vi "DisplayDataChartDialog.vi"(8 "Error In":errorcluster) -> (0 "Error Out":errorcluster)   [LabVIEW 2012]
uses:
  DisplayDataChartAction.ctl
  <vilib>/Platform/TimedLoop/XDataNode/timing_clust.ctl
  <vilib>/Platform/TimedLoop/XDataNode/nitl_modes.ctl
  <vilib>/Platform/TimedLoop/XDataNode/wakeup.ctl
  DisplayDataGlobalAction.ctl
  <vilib>/platform/TimedLoop/XDataNode/XDataNode.xnode
  <vilib>/Platform/TimedLoop/XDataNode/XDNodeRunTimeDep.lvlib
panel:
  in  "RESET":bool
  in  "Live DUT":u32=1 min=1 step=1
  in  "Live SMU":enum16{"A", "B"}(ring)
  in  "Live Measure Value":enum16{"Voltage", "Current", "Resistance"}(ring)
  out "Live SMU Value":dbl format="%_4p"
  out "Live SMU Units":enum16{"V", "A", "Ohm"}(ring)
  out "Live SMU Chart":dbl(graph)
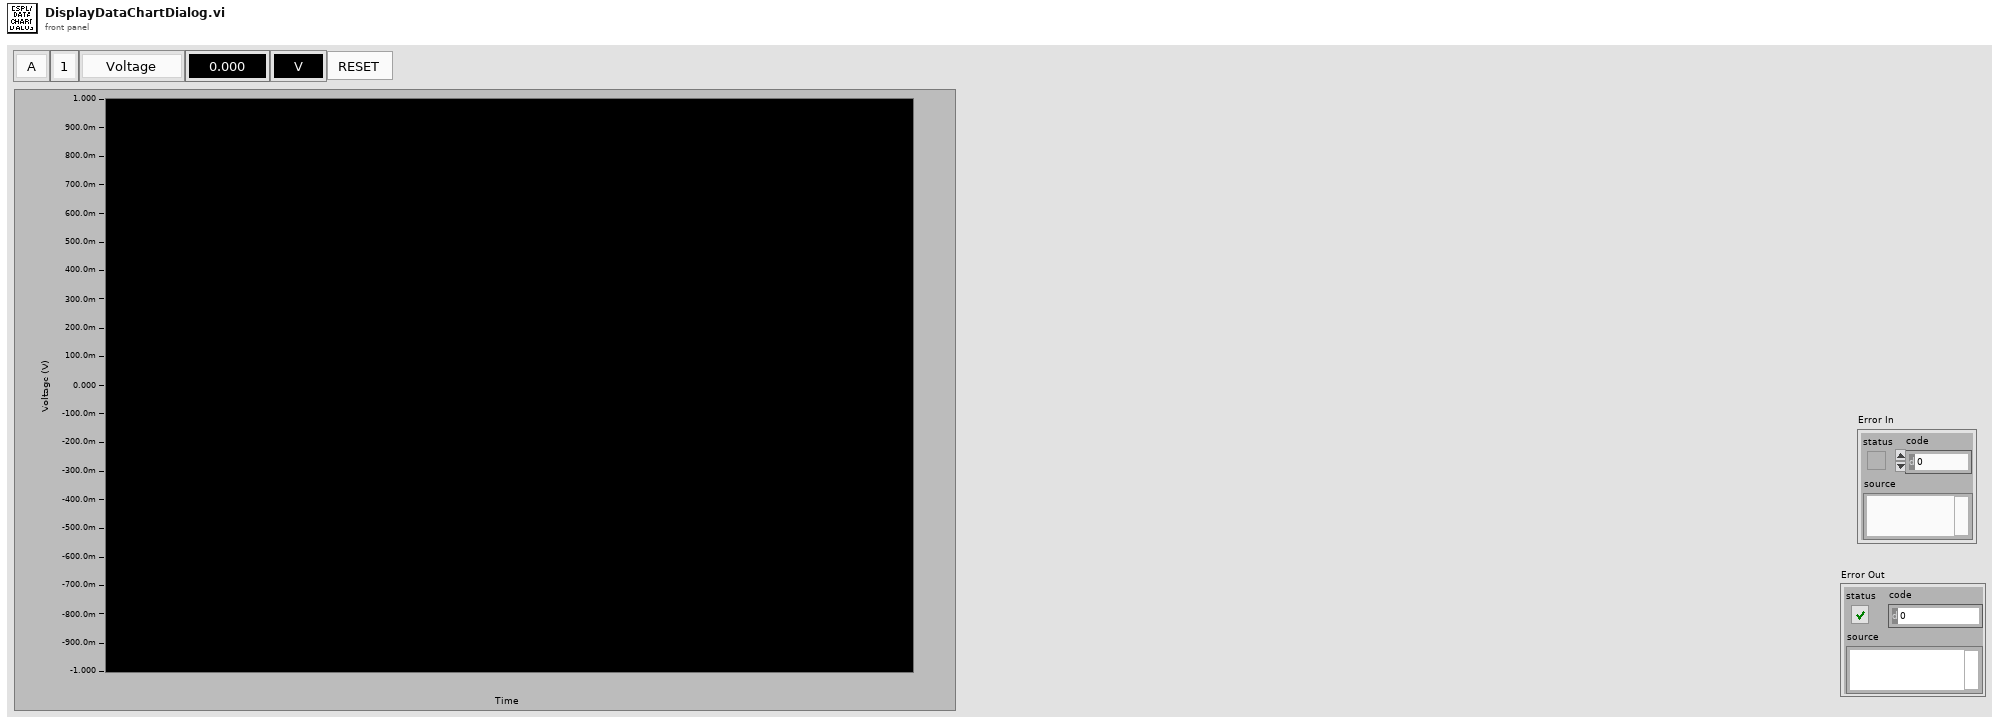
[diagram p1: front panel]
types:
  T1 = typedef "DisplayDataGlobalAction.ctl" = enum16{"Get", "Set"}
  T2 = typedef "XDNodeRunTimeDep.lvlib/timing_clust.ctl" = cluster{"Expected End [f-1]":u64, "Actual End [f-1]":u64, "Finished Late? [f-1]":bool, "Expected End [i-1]":u64, "Actual End [i-1]":u64, "Finished Late? [i-1]":bool, "Expected Start [i]":u64, "Actual Start [i]":u64, "Expected Start [f]":u64, "Actual Start [f]":u64, "Source Name":string, "Structure Name":string, "Period":i64, "Deadline":i64, "Offset":i64, "Start":i64, "Priority":i32, "Timeout":i32, "Mode":T3, "Wakeup Reason":T4, "Error":errorcluster, "Source Type":string, "Secondary Source Type":string, "Global End Time":u64, "Global Start Time":u64, "Frame Duration":u64, "Iteration Duration":u64, "Assigned CPU":i32, "I/O Scan Engine Mode":u32}
  T3 = typedef "XDNodeRunTimeDep.lvlib/nitl_modes.ctl" = enum32{"No Change", "Process missed periods, maintain original phase", "Discard missed periods, maintain original phase", "Process missed periods, ignore original phase", "Discard missed periods, ignore original phase"}
  T4 = typedef "XDNodeRunTimeDep.lvlib/wakeup.ctl" = enum32{"Normal", "Aborted", "Asynchronous wakeup", "Timing source error", "Timed loop error", "Timeout"}
  T5 = typedef "DisplayDataChartAction.ctl" = enum16{"Initialize", "Shutdown", "Update", "Reset"}
  T6 = cluster{"Live SMU":enum16{"A", "B"}, "Live DUT":u32, "Live Measure Value":enum16{"Voltage", "Current", "Resistance"}}
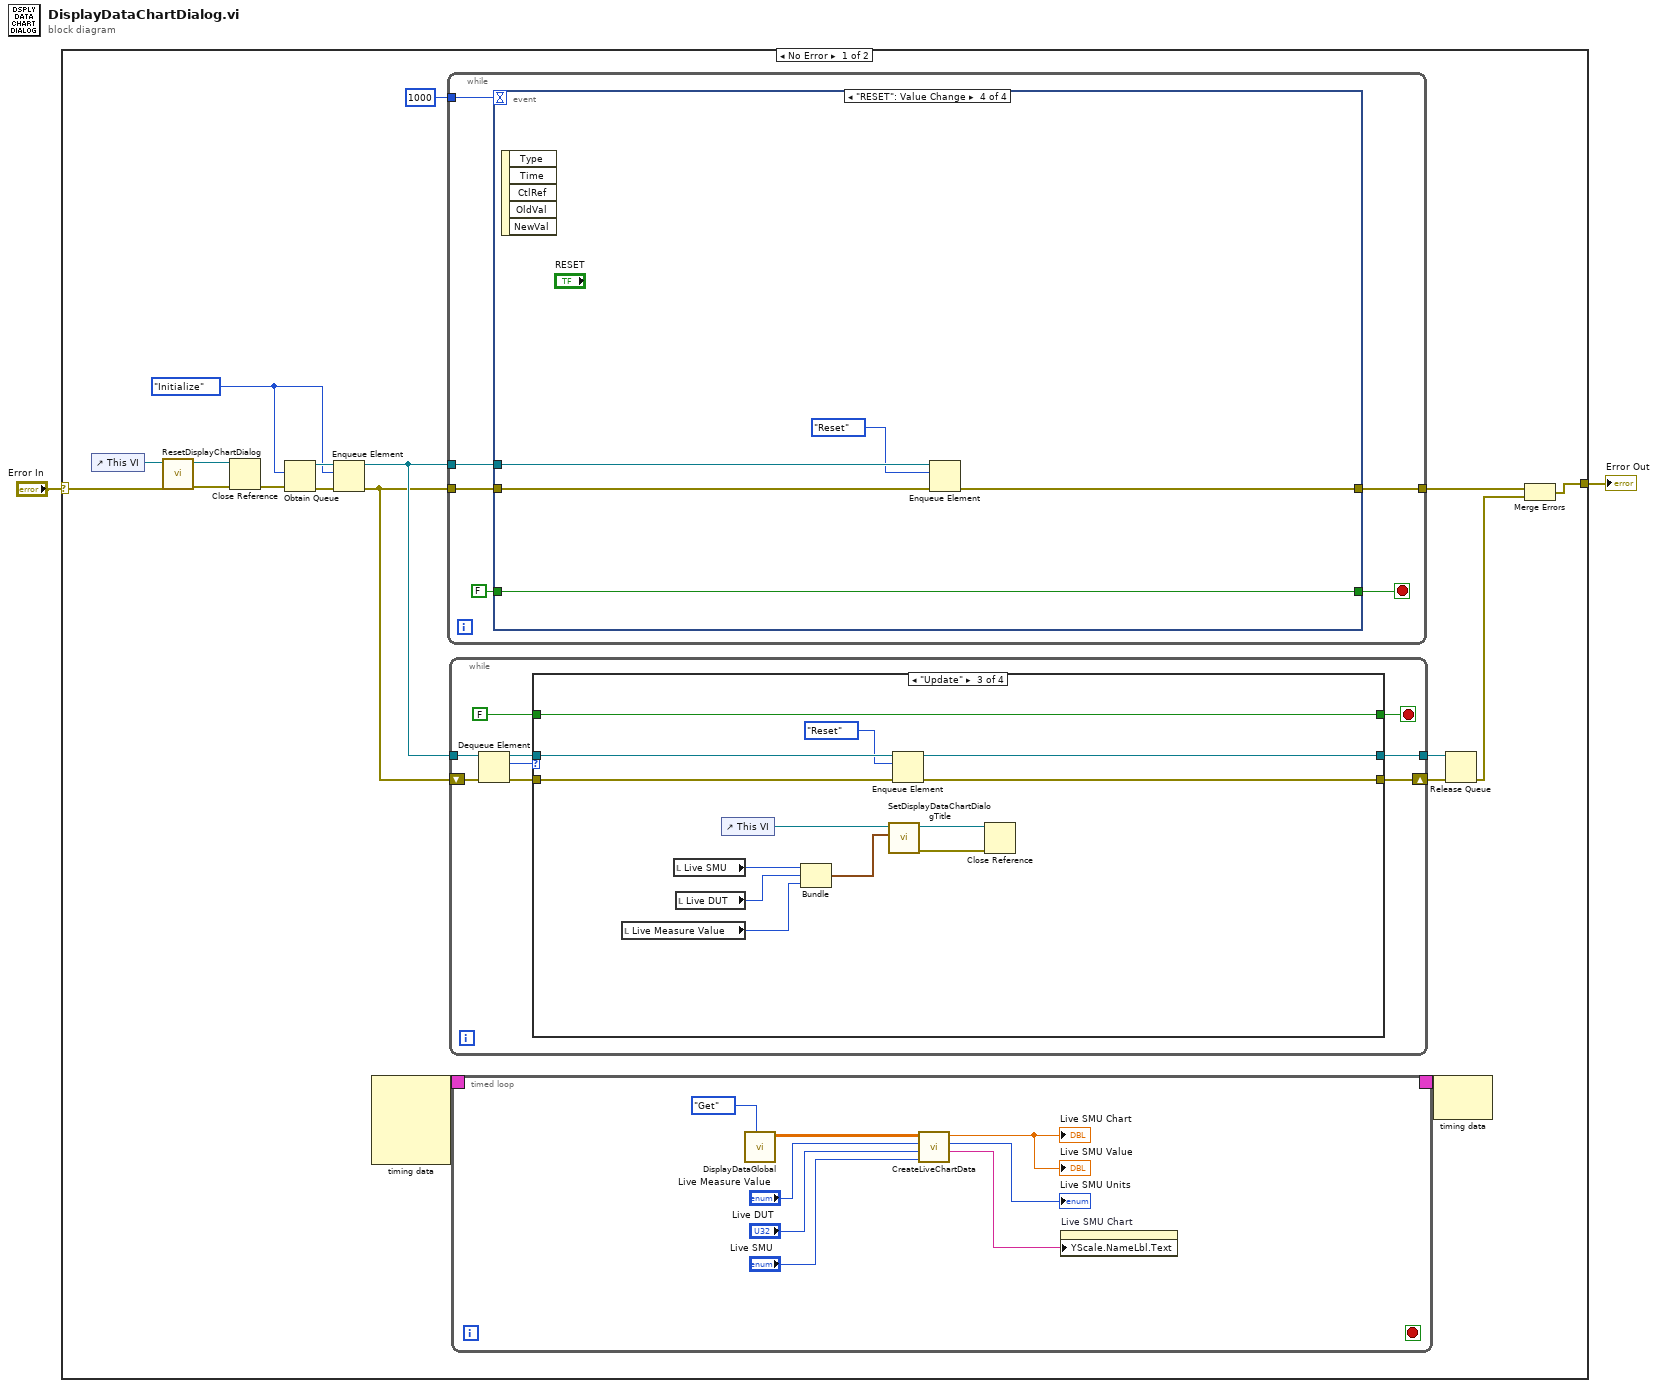
[diagram p0: block diagram]
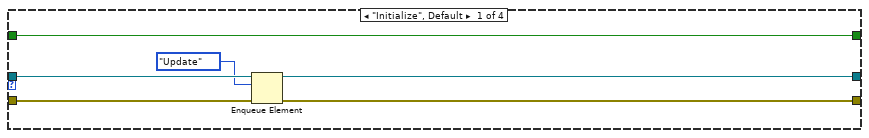
[diagram p2: hidden frame]
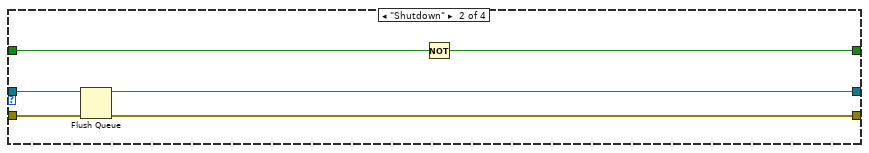
[diagram p3: hidden frame]
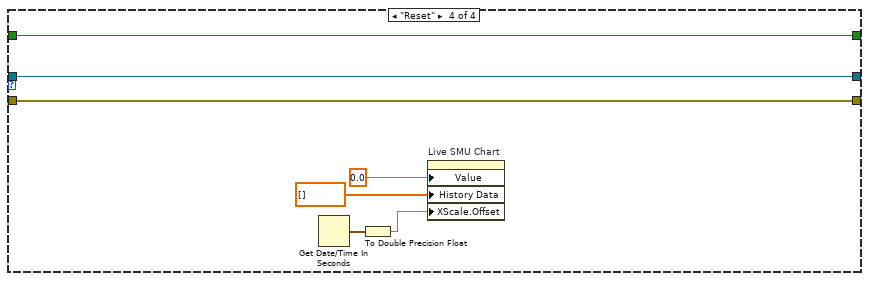
[diagram p4: hidden frame]
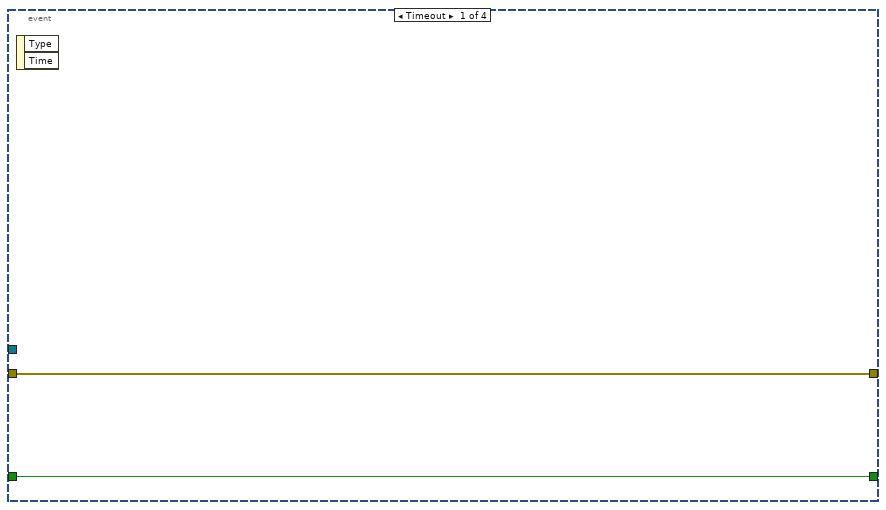
[diagram p5: hidden frame]
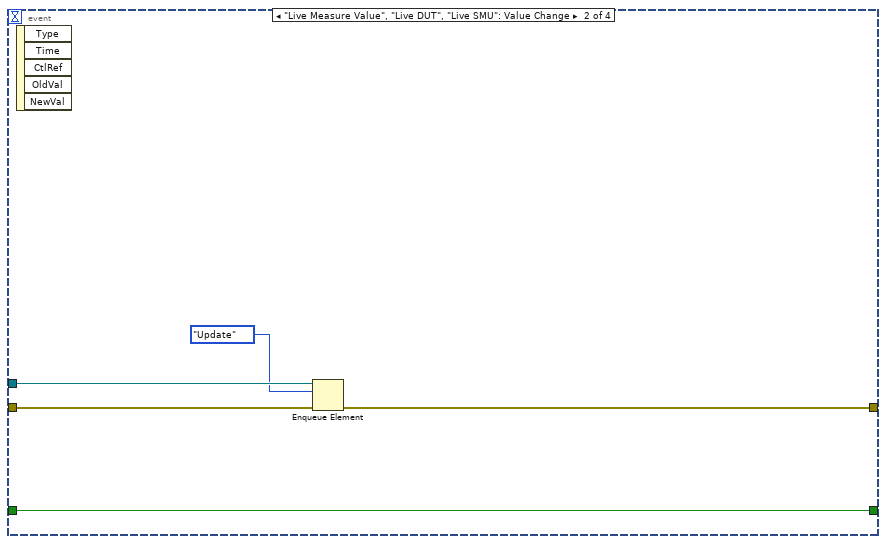
[diagram p6: hidden frame]
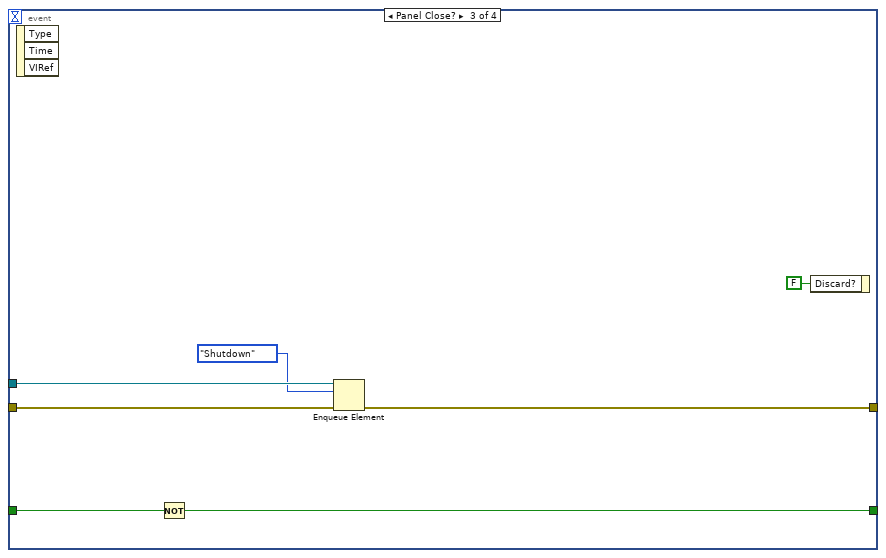
[diagram p7: hidden frame]
diagram:
  n1 = case shown="No Error" "Error In" {
    selector: "Error In" -> [w3 w99]
    tunnel: [w11 w99] -> w1
    frame No Error {
      w15 = DisplayDataChartAction."Initialize" ("Action")
      n2 = control-ref of="This VI"() -> (w4:refnum<vi>)
      n3 = call "ResetDisplayChartDialog.vi"("Error In"=w3, "VI Ref In"=w4) -> ("Error Out"=w6:errorcluster, "VI Ref Out"=w7:refnum<vi>)  [unwired: 8 in]
      n4 = Close Reference(reference=w7, error in (no error)=w6) -> (error out=w5:errorcluster)
      n5 = Obtain Queue(element data type=w15, error in (no error)=w5) -> (queue out=w17:refnum<queue>, error out=w16:errorcluster)  [unwired: 3 in, 1 out]
      n6 = Enqueue Element(queue=w17, element=w15, error in (no error)=w16) -> (queue out=w14:refnum<queue>, error out=w13:errorcluster)  [unwired: 1 in, 1 out]
      n7 = node-c288() -> (w19:T2)  [unwired: 4 in]
      n8 = while {
        tunnel: 1000 -> [w77]
        tunnel: w14 -> [w76]
        tunnel: w13 -> [w75]
        tunnel: [w74] -> w12
        stop <- w78 stop-if-true
        n9 = event shown="[3] \"RESET\": Value Change" {
          selector: _ -> [_ _ _ _]
          dyn-events: _ -> [_ _ _ _]
          timeout: w77 -> [_ _ _ _]
          tunnel: FALSE -> [w81 w86 w90 w98]
          tunnel: [w81 w86 w89 w98] -> w78
          tunnel: w76 -> [_ w84 w92 w95]
          tunnel: w75 -> [w80 w85 w91 w97]
          tunnel: [w80 w82 w88 w96] -> w74
          event Timeout {
            n10 = event-data() -> ()  [unwired: 1 in, 2 out]
          }
          event "Live Measure Value", "Live DUT", "Live SMU": Value Change {
            n11 = event-data() -> ()  [unwired: 1 in, 5 out]
            n12 = Enqueue Element(queue=w84, element=DisplayDataChartAction."Update", error in (no error)=w85) -> (error out=w82:errorcluster)  [unwired: 1 in, 2 out]
          }
          event Panel Close? {
            n13 = event-data() -> ()  [unwired: 1 in, 3 out]
            n14 = Not(x=w90) -> (.not. x?=w89:bool)
            n15 = Enqueue Element(queue=w92, element=DisplayDataChartAction."Shutdown", error in (no error)=w91) -> (error out=w88:errorcluster)  [unwired: 1 in, 2 out]
            n16 = event-data("Discard?"=FALSE) -> ()  [unwired: 1 in, 1 out]
          }
          event "RESET": Value Change {
            n17 = event-data() -> ()  [unwired: 1 in, 5 out]
            n18 = Enqueue Element(queue=w95, element=DisplayDataChartAction."Reset", error in (no error)=w97) -> (error out=w96:errorcluster)  [unwired: 1 in, 2 out]
          }
        }
      }
      n19 = while {
        tunnel: w14 -> [w39]
        shift-right: [w34] -> w9
        shift-left: w13 -> [w38]
        tunnel: [w33] -> w10
        stop <- w40 stop-if-true
        n20 = Dequeue Element(queue=w39, error in (no error)=w38) -> (queue out=w36:refnum<queue>, element=w37:T5, error out=w35:errorcluster)  [unwired: 1 in, 1 out]
        n21 = case shown="\"Update\"" w37 {
          tunnel: FALSE -> [w47 w53 w66 w68]
          tunnel: [w47 w52 w66 w68] -> w40
          tunnel: w36 -> [w46 w51 w65 w67]
          tunnel: w35 -> [w45 w50 w64 w69]
          tunnel: [w44 w49 w63 w69] -> w34
          tunnel: [w42 w48 w61 w67] -> w33
          frame "Initialize", Default {
            n22 = Enqueue Element(queue=w46, element=DisplayDataChartAction."Update", error in (no error)=w45) -> (queue out=w42:refnum<queue>, error out=w44:errorcluster)  [unwired: 1 in, 1 out]
          }
          frame "Shutdown" {
            n23 = Flush Queue(queue=w51, error in (no error)=w50) -> (queue out=w48:refnum<queue>, error out=w49:errorcluster)  [unwired: 1 out]
            n24 = Not(x=w53) -> (.not. x?=w52:bool)
          }
          frame "Update" {
            n25 = local read "Live Measure Value"() -> (w55:enum16{"Voltage", "Current", "Resistance"})
            n26 = local read "Live SMU"() -> (w57:enum16{"A", "B"})
            n27 = local read "Live DUT"() -> (w56:u32)
            n28 = control-ref of="This VI"() -> (w60:refnum<vi>)
            n29 = Bundle("Live SMU"=w57, "Live DUT"=w56, "Live Measure Value"=w55) -> (w54:T6)  [unwired: 1 in]
            n30 = call "SetDisplayDataChartDialogTitle.vi"("Chart Settings"=w54, "VI Ref In"=w60) -> ("Error Out"=w58:errorcluster, "VI Ref Out"=w59:refnum<vi>)  [unwired: 8 in]
            n31 = Enqueue Element(queue=w65, element=DisplayDataChartAction."Reset", error in (no error)=w64) -> (queue out=w61:refnum<queue>, error out=w63:errorcluster)  [unwired: 1 in, 1 out]
            n32 = Close Reference(reference=w59, error in (no error)=w58) -> ()  [unwired: 1 out]
          }
          frame "Reset" {
            n33 = Get Date/Time In Seconds() -> (seconds since 1Jan1904=w72:timestamp)
            n34 = To Double Precision Float(number=w72) -> (double precision float=w73:dbl)
            n35 = property on="Live SMU Chart" class="WFChart (strict)"("Value"=0.0 ("Chart"), "History Data"=dbl[] [], "XScale.Offset"=w73) -> ()  [unwired: 2 in, 2 out]
          }
        }
      }
      n36 = timed-loop {
        timing: w19 -> [_]
        timing-out: [_] -> w18
        stop <- _ stop-if-true
        n37 = call "DisplayDataGlobal.vi"("Action"=DisplayDataGlobalAction."Get") -> ("Value Out"=w27:dbl[][])  [unwired: 10 in]
        n38 = call "CreateLiveChartData.vi"("Live SMU"="Live SMU", "Live DUT"="Live DUT", "Live Measure Value"="Live Measure Value", "SMU"=w27) -> ("Live SMU Chart Y Scale Name"=w22:string, "Live SMU Units"=→"Live SMU Units":enum16{"V", "A", "Ohm"}, "Live SMU Chart"=→"Live SMU Chart" →"Live SMU Value":dbl)  [unwired: 5 in]
        n39 = property on="Live SMU Chart" class="WFChart (strict)"("YScale.NameLbl.Text"=w22) -> ()  [unwired: 2 in, 2 out]
      }
      n40 = node-c288(w18) -> ()  [unwired: 1 out]
      n41 = Release Queue(queue=w10, error in (no error)=w9) -> (error out=w8:errorcluster)  [unwired: 1 in, 2 out]
      n42 = Merge Errors(w12, w8) -> (w11:errorcluster)
    }
    frame Error {
    }
  }
  "Error Out" <- w1
